vi "Extract Unique IDs.vi"(0 "Data":string[][](array[string]), 9 "Stats":string[][](array[string]), 13 "Test Style":enum32{"Flow", "Test", "Hot\nFuel"}(ring)) -> (4 "Data with IDs":string[][](array[string]), 10 "Stats with IDs":string[][](array[string]))   [LabVIEW 2013]
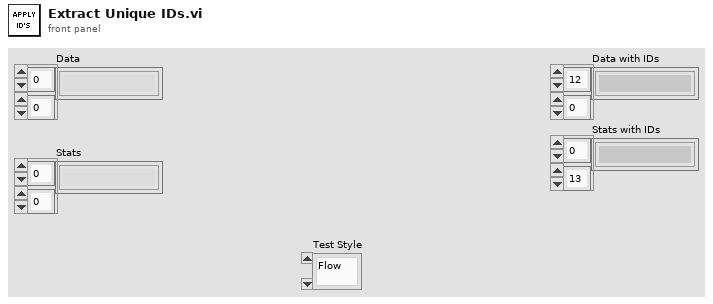
[diagram p1: front panel]
types:
  T1 = cluster{"disabled index (col)":i32, string[], string[]}
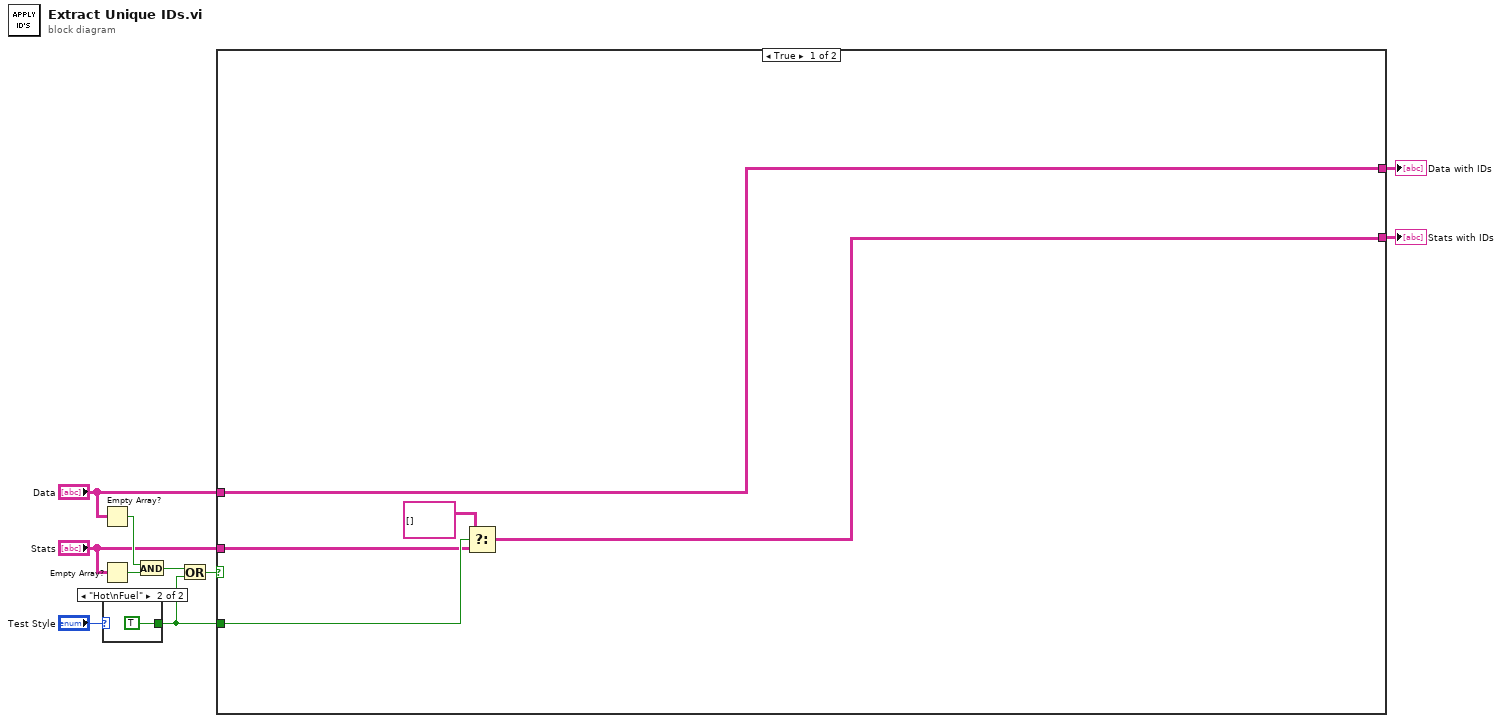
[diagram p0: block diagram]
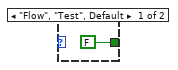
[diagram p2: hidden frame]
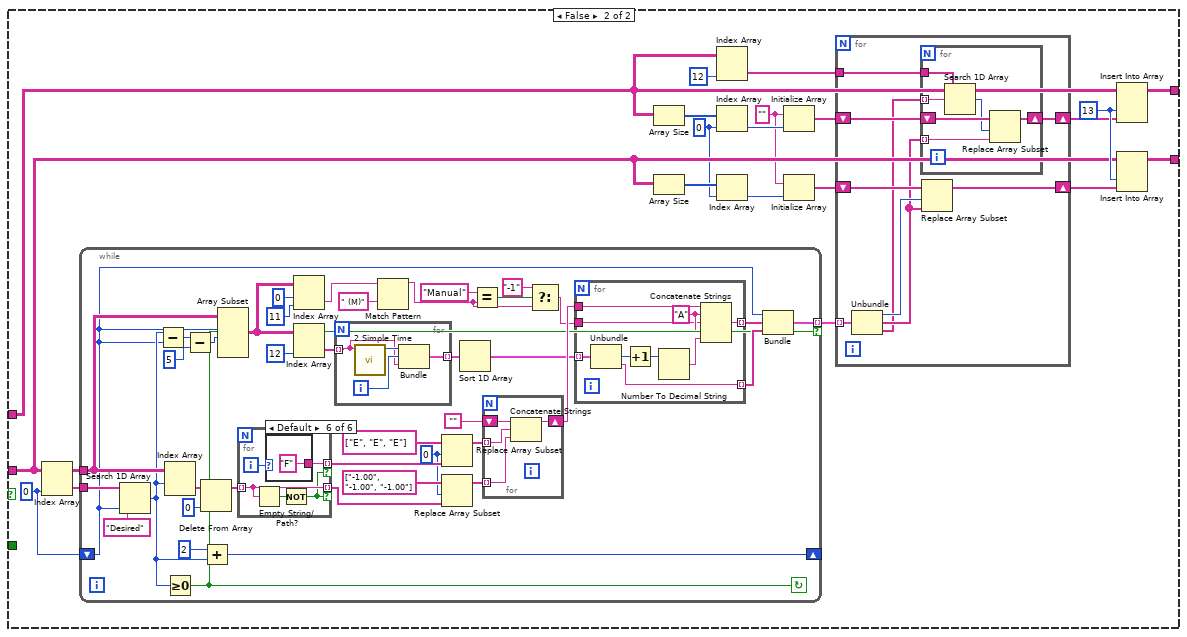
[diagram p3: hidden frame]
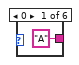
[diagram p4: hidden frame]
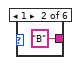
[diagram p5: hidden frame]
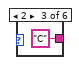
[diagram p6: hidden frame]
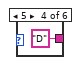
[diagram p7: hidden frame]
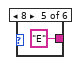
[diagram p8: hidden frame]
diagram:
  n1 = Empty Array?(array="Data") -> (empty?=w10:bool)
  n2 = Empty Array?(array="Stats") -> (empty?=w9:bool)
  n3 = case shown="\"Hot\\nFuel\"" "Test Style" {
    tunnel: [FALSE TRUE] -> w1
    frame "Flow", "Test", Default {
    }
    frame "Hot\nFuel" {
    }
  }
  n4 = And(x=w10, y=w9) -> (x .and. y?=w3:bool)
  n5 = Or(x=w3, y=w1) -> (x .or. y?=w2:bool)
  n6 = case shown="True" w2 {
    tunnel: "Data" -> [w17 w20]
    tunnel: "Stats" -> [w14 w33]
    tunnel: [w17 w18] -> w6
    tunnel: [w13 w21] -> w5
    tunnel: w1 -> [w16 _]
    frame True {
      n7 = Select(t=string[][] [], s=w16, f=w14) -> (s? t:f=w13:string[][])
    }
    frame False {
      w26 = 0 ("index")
      w28 = ""
      w35 = 13 ("disabled index (col)")
      w36 = 0 ("disabled index (col)")
      n8 = Index Array(array=w33, index (col)=w36) -> (element=w37:string[])  [unwired: 1 in]
      n9 = while {
        tunnel: w37 -> [w92]
        tunnel: w33 -> [w77]
        shift-right: [w89] -> _
        shift-left: w36 -> [w67]
        tunnel: [w64] -> w34 mode=indexing if=w63
        stop <- w63 continue-if-true
        w82 = 0 ("index")
        n10 = Search 1D Array(1D array=w92, element="Desired", start index (0)=w67) -> (index of element=w76:i32)
        n11 = Subtract(x=w76, y=w67) -> (x-y=w62:i32)
        n12 = Index Array(array=w77, index (row)=w76) -> (element=w88:string[])  [unwired: 1 in]
        n13 = Greater Or Equal To 0?(x=w76) -> (x >= 0?=w63:bool)
        n14 = Subtract(x=w62, y=5) -> (x-y=w61:i32)
        n15 = Delete From Array(array=w88, index=0) -> (array with subset deleted=w86:string[])  [unwired: 1 in, 1 out]
        n16 = Add(x=2, y=w76) -> (x+y=w89:i32)
        n17 = Array Subset(array=w77, index (row)=w67, length (row)=w61) -> (w72:string[][])  [unwired: 2 in]
        n18 = for {
          tunnel: w86 -> [w114] mode=indexing
          tunnel: [w110] -> w84 mode=indexing if=w112
          tunnel: [w114] -> w81 mode=indexing if=w112
          i -> [w111]
          n19 = Empty String/Path?(string/path=w114) -> (empty?=w113:bool)
          n20 = case shown="Default" w111 {
            tunnel: ["A" "B" "C" "D" "E" "F"] -> w110
            frame 0 {
            }
            frame 1 {
            }
            frame 2 {
            }
            frame 5 {
            }
            frame 8 {
            }
            frame Default {
            }
          }
          n21 = Not(x=w113) -> (.not. x?=w112:bool)
        }
        n22 = Index Array(array=w72, index (row)=0, index (col)=11 ("disabled index (col)")) -> (element=w58:string)
        n23 = Index Array(array=w72, index (col)=12 ("disabled index (col)")) -> (element=w74:string[])  [unwired: 1 in]
        n24 = for {
          tunnel: w74 -> [w102] mode=indexing
          tunnel: [w103] -> w73 mode=indexing
          i -> [w104]
          n25 = call "2 Simple Time.vi"("Timestamp"=w102) -> ("Simple Time"=w105:i64)  [unwired: 9 in, 1 out]
          n26 = Bundle("Simple Time"=w105, w104, w102) -> (w103:cluster{"Simple Time":i64, i32, string})  [unwired: 1 in]
        }
        n27 = Match Pattern(string=w58, regular expression=" (M)") -> (before substring=w55:string)  [unwired: 1 in, 3 out]
        n28 = Replace Array Subset(array=string[] ["E", "E", "E"], new element=w84, index=w82) -> (w80:string[])
        n29 = Replace Array Subset(array=string[] ["-1.00", "-1.00", "-1.00"], new element=w81, index=w82) -> (w79:string[])
        n30 = Sort 1D Array(array=w73) -> (sorted array=w68:cluster{"Simple Time":i64, i32, string}[])
        n31 = Equal?(x="Manual", y=w55) -> (x = y?=w56:bool)
        n32 = for {
          tunnel: w80 -> [w107] mode=indexing
          tunnel: w79 -> [w106] mode=indexing
          shift-right: [w108] -> w69
          shift-left: "" -> [w109]
          n33 = Concatenate Strings(w109, w107, w106) -> (w108:string)
        }
        n34 = Select(t="-1", s=w56, f=w55) -> (s? t:f=w53:string)
        n35 = for {
          tunnel: w69 -> [w99]
          tunnel: w68 -> [w101] mode=indexing
          tunnel: w53 -> [w97]
          tunnel: [w94] -> w66 mode=indexing
          tunnel: [w93] -> w65 mode=indexing
          w98 = "A" ("string")
          n36 = Unbundle(w101) -> (w100:i32, w93:string)  [unwired: 1 out]
          n37 = Increment(x=w100) -> (x+1=w96:i32)
          n38 = Number To Decimal String(number=w96) -> (decimal integer string=w95:string)  [unwired: 1 in]
          n39 = Concatenate Strings(w99, w98, w97, w98, w95) -> (w94:string)
        }
        n40 = Bundle("disabled index (col)"=w67, w66, w65) -> (w64:T1)  [unwired: 1 in]
      }
      n41 = Array Size(array=w20) -> (size(s)=w32:i32[])
      n42 = Array Size(array=w33) -> (size(s)=w31:i32[])
      n43 = Index Array(array=w20, index (col)=12 ("disabled index (col)")) -> (element=w22:string[])  [unwired: 1 in]
      n44 = Index Array(array=w32, index=w26) -> (element=w30:i32)
      n45 = Index Array(array=w31, index=w26) -> (element=w29:i32)
      n46 = Initialize Array(w28, w30) -> (w27:string[])
      n47 = Initialize Array(w28, w29) -> (w25:string[])
      n48 = for {
        tunnel: w34 -> [w46] mode=indexing
        shift-right: [w38] -> w19
        shift-left: w27 -> [w42]
        shift-right: [w43] -> w24
        shift-left: w25 -> [w45]
        tunnel: w22 -> [w39]
        n49 = Unbundle(w46) -> ("disabled index (col)"=w44:i32, w41:string[], w40:string[])
        n50 = for {
          shift-right: [w49] -> w38
          shift-left: w42 -> [w50]
          tunnel: w41 -> [w47] mode=indexing
          tunnel: w40 -> [w51] mode=indexing
          tunnel: w39 -> [w52]
          n51 = Search 1D Array(1D array=w52, element=w51) -> (index of element=w48:i32)  [unwired: 1 in]
          n52 = Replace Array Subset(array=w50, new element=w47, index=w48) -> (w49:string[])
        }
        n53 = Replace Array Subset(array=w45, new element=w41, index=w44) -> (w43:string[])
      }
      n54 = Insert Into Array(array=w20, index (col)=w35, new element=w19) -> (w18:string[][])  [unwired: 1 in]
      n55 = Insert Into Array(array=w33, index (col)=w35, new element=w24) -> (w21:string[][])  [unwired: 1 in]
    }
  }
  "Data with IDs" <- w6
  "Stats with IDs" <- w5
